vi "configuration UI.vi"() -> ()   [LabVIEW 2013, in "TDMS datalogger editor node.lvclass"]
uses:
  TDMS datalogger editor node.lvclass
  <vilib>/NI/Configuration Framework/Node/NodeRef.ctl
  <vilib>/NI/Configuration Framework/Node/NISE_CEF_Node.lvclass
  <vilib>/NI/AMC/Message Queue.ctl
  <vilib>/NI/AMC/Message.ctl
  <vilib>/NI/Tools/Keyed Array/KeyedArray.ctl
  <vilib>/NI/Configuration Framework/Node/UserEventRef.ctl
  <vilib>/NI/Configuration Framework/Controls/EventCluster.ctl
  module/configuration/TDMS datalogger configuration.lvclass
  <vilib>/NI/Tag Bus Data Framework/Configuration Editor/Classes/Engine Parent/Engine Parent Editor Node.lvclass
  <vilib>/NI/Tag Bus/tag/tag descriptor.lvclass
  <vilib>/NI/Tag Bus/tag/Data Type.ctl
  <vilib>/NI/Module Execution Interface/Engine Configuration/engine configuration.lvclass
  <vilib>/NI/Tag Bus/tag/tag descriptor.lvclass/tag descriptor.ctl
  <vilib>/NI/Configuration Framework/serializable configuration/NISE_CEF_serializable configuration.lvclass/NISE_CEF_serializable configuration.ctl
  <vilib>/NI/Configuration Framework/serializable configuration/NISE_CEF_serializable configuration.lvclass
  module/configuration/TDMS datalogger configuration.lvclass/TDMS datalogger configuration.ctl
  TDMS datalogger editor node.lvclass/TDMS datalogger editor node.ctl
  <vilib>/NI/Tag Bus/tag/write tag name.vi
  <vilib>/NI/Tag Bus/tag/write data type.vi
  module/configuration/Write scans per write.vi
  module/configuration/Write queue size.vi
  module/configuration/Write Path.vi
  module/configuration/Write backup directory.vi
  module/configuration/Write channel pattern matches.vi
  <vilib>/NI/Configuration Framework/serializable configuration/Read UID.vi
  module/configuration/Read backup directory.vi
  module/configuration/Read Path.vi
  module/configuration/Read queue size.vi
  module/configuration/Read scans per write.vi
  module/configuration/Read add enable channel.vi
  module/configuration/Read channel pattern matches.vi
  <vilib>/NI/Tag Bus Data Framework/Configuration Editor/Classes/Module editor node/Read Module Configuration.vi
  <vilib>/NI/Tag Bus Module Framework/module configuration/TBM module configuration.lvclass
  <vilib>/NI/Tag Bus Data Framework/Configuration Editor/Classes/Module editor node/module editor node.lvclass
  <vilib>/NI/Configuration Framework/NISE_CEF_TreeControl.lvlib
  <vilib>/NI/Tools/Keyed Array/Tools_KeyedArray.lvlib
  <vilib>/NI/AMC/AMC.lvlib
panel:
  in  "Tab Control":T1(tab)
  in  "channels":i32(listbox)
  in  "remove":bool
  in  "avail tags":i32(listbox)=-1
  in  "add all":bool
  in  "add1":bool
  out "Enable Tag":string
  in  "history error":bool
  in  "path error":bool
  in  "Historical Directory":path
  in  "use enable channel":bool
  in  "recalc":bool
  out "Approximate memory usage":dbl
  in  "queue size":i32=2
  in  "scans per write":i32=20
  in  "File Path":path
  in  "Channel Subscription Pattern Matches":string[](array[string])
  in  "Enable Dynamic Mapping":bool
  in  "user event":T2
  in  "main queue":T3
  in  "node ref":T4
  # "kB"
  # "Note: This value ignores dynamic mapping"
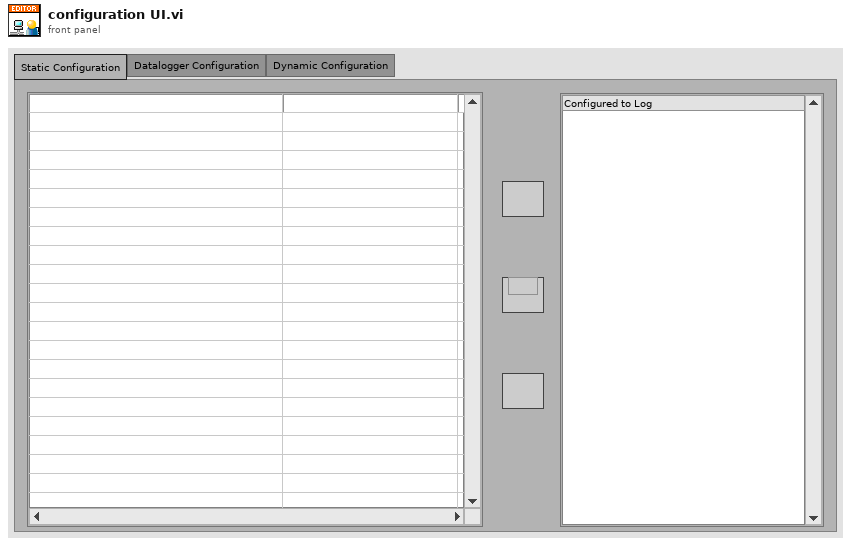
[diagram p1: front panel]
types:
  T1 = enum32{"Static Configuration", "Datalogger Configuration", "Dynamic Configuration"}
  T2 = typedef "NISE_CEF_Node.lvclass/UserEventRef.ctl" = refnum<user-event>
  T3 = typedef "AMC.lvlib/Message Queue.ctl" = refnum<queue>
  T4 = typedef "NISE_CEF_Node.lvclass/NodeRef.ctl" = refnum<data-value>
  T5 = typedef "NISE_CEF_TreeControl.lvlib/EventCluster.ctl" = cluster{"command":string, "data":string}
  T6 = typedef "tag bus.lvlib/tag descriptor.lvclass/Data Type.ctl" = enum16{"Double", "Single", "I64", "I32", "I16", "I8", "U64", "U32", "U16", "U8", "Boolean", "String", "Array of Double", "Array of Single", "Array of I64", "Array of I32", "Array of I16", "Array of I8", "Array of U64", "Array of U32", "Array of U16", "Array of U8", "Array of Boolean", "Array of String"}
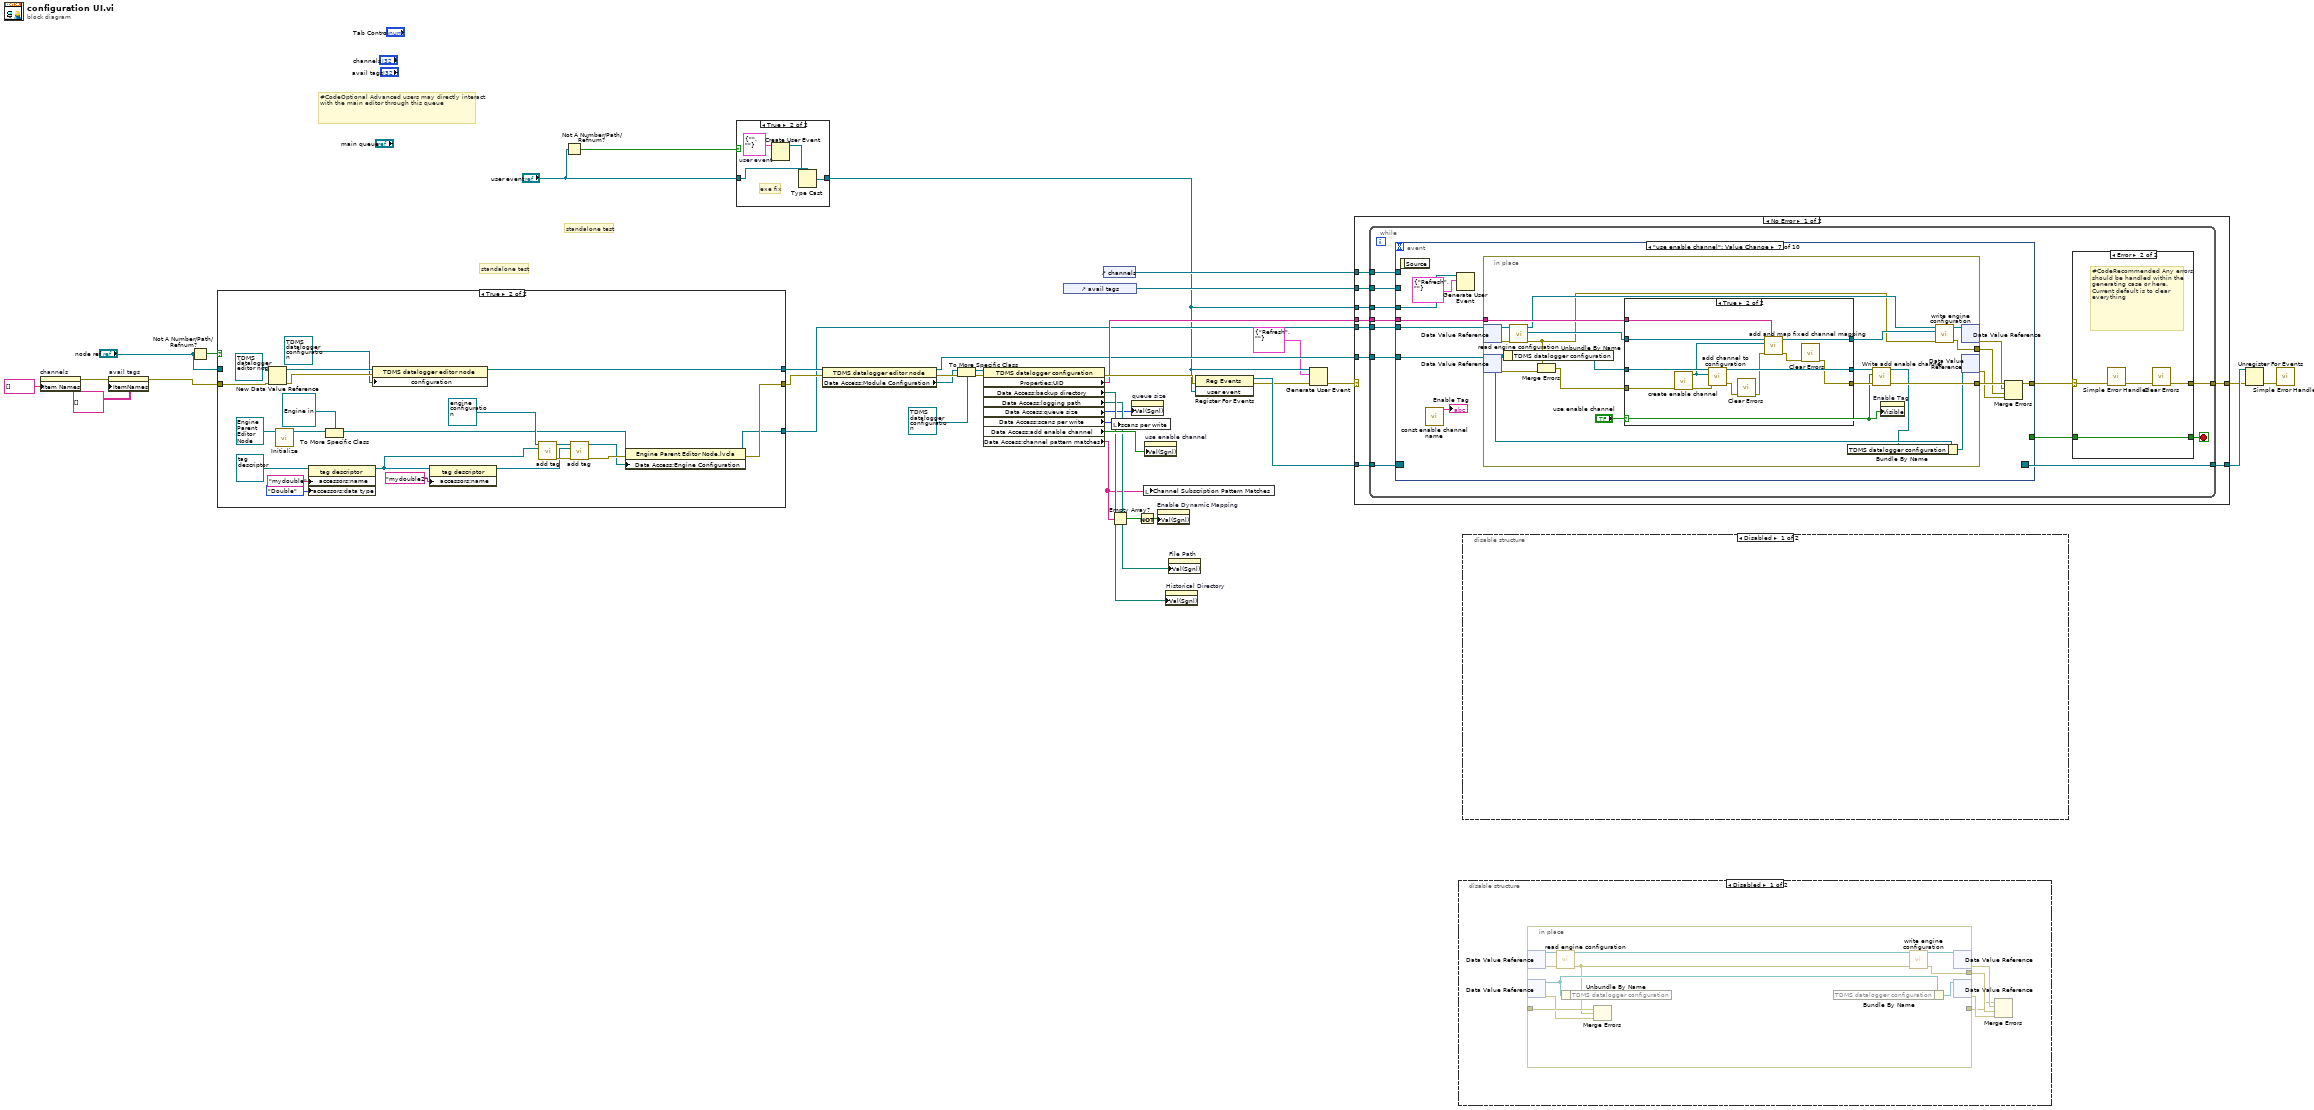
[diagram p0: block diagram]
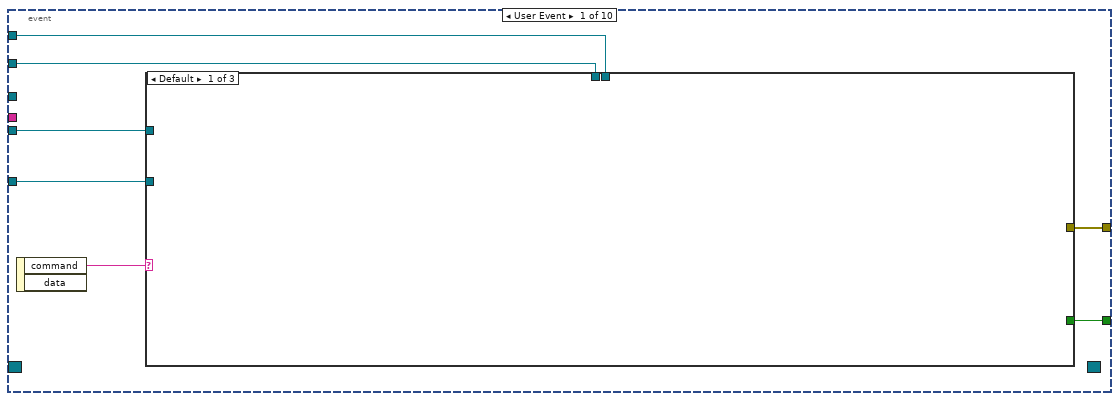
[diagram p4: hidden frame]
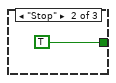
[diagram p5: hidden frame]
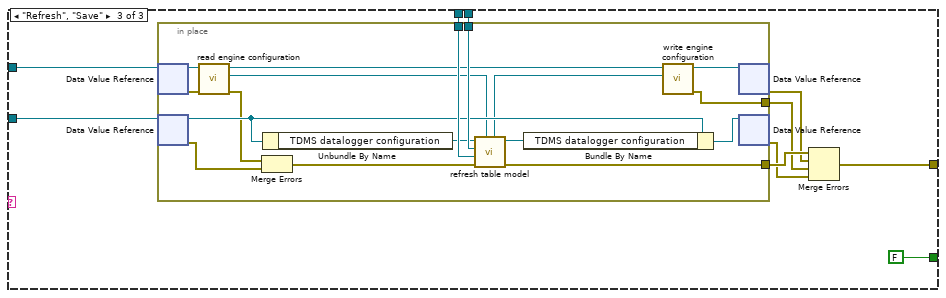
[diagram p6: hidden frame]
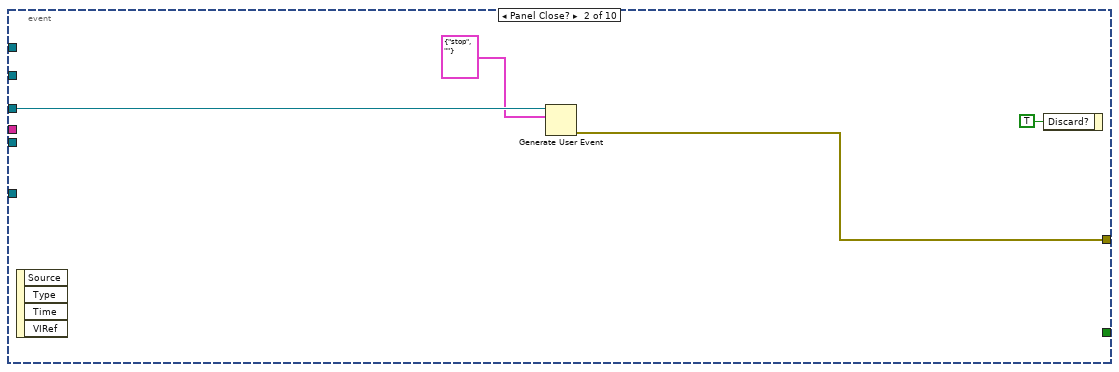
[diagram p7: hidden frame]
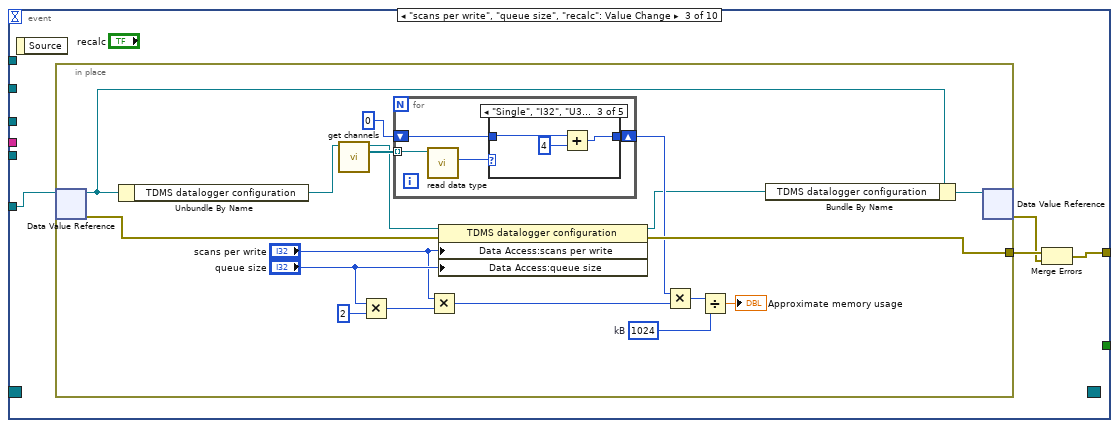
[diagram p8: hidden frame]
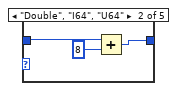
[diagram p10: hidden frame]
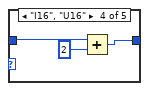
[diagram p11: hidden frame]
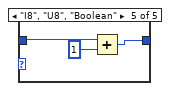
[diagram p12: hidden frame]
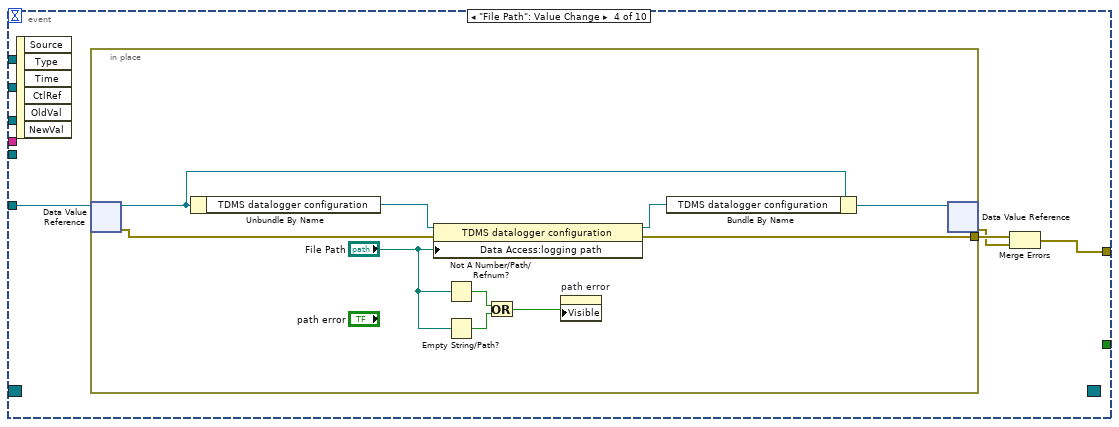
[diagram p13: hidden frame]
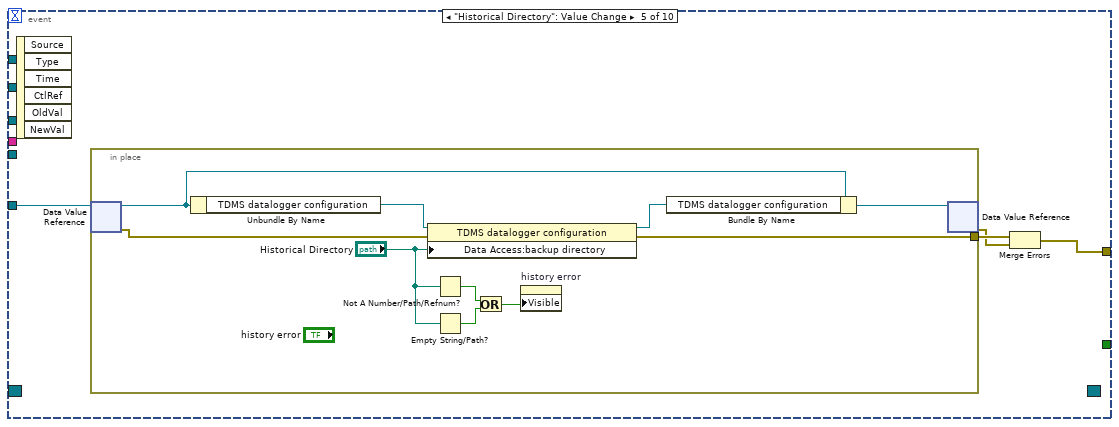
[diagram p14: hidden frame]
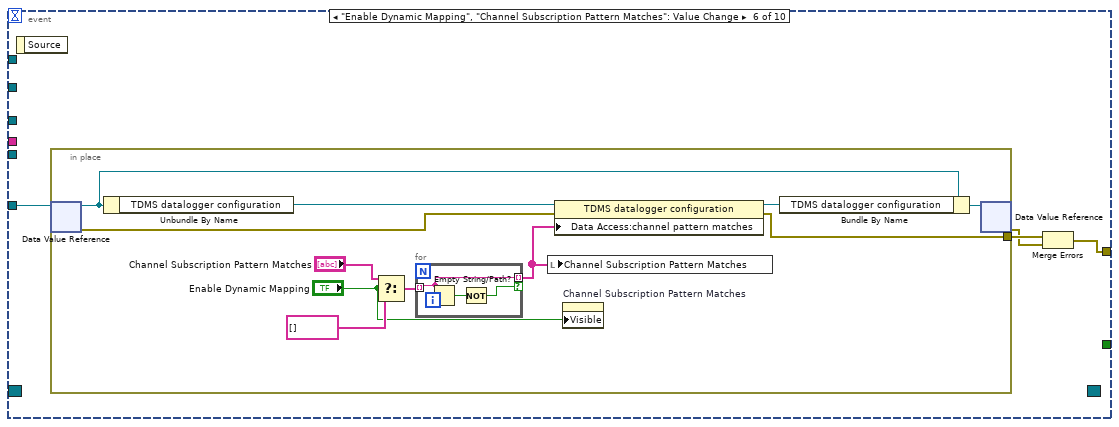
[diagram p15: hidden frame]
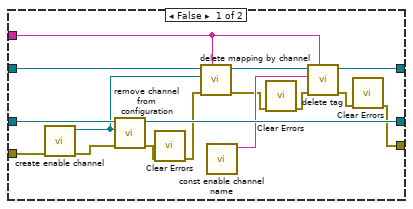
[diagram p16: hidden frame]
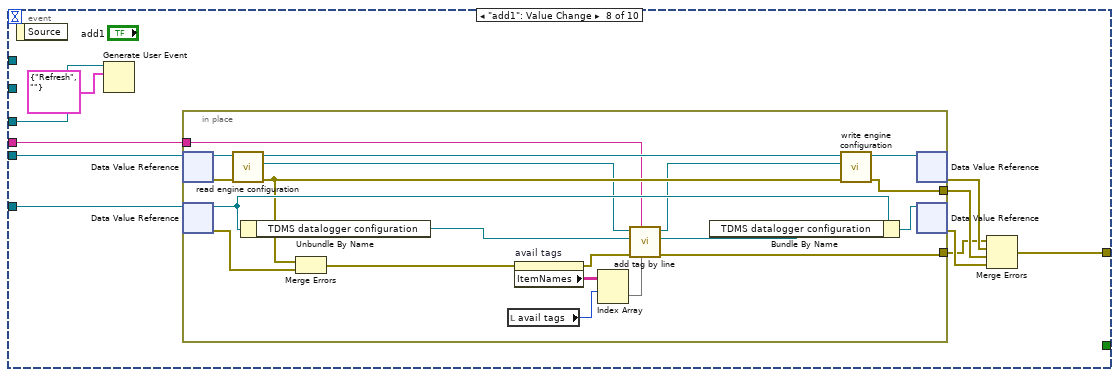
[diagram p17: hidden frame]
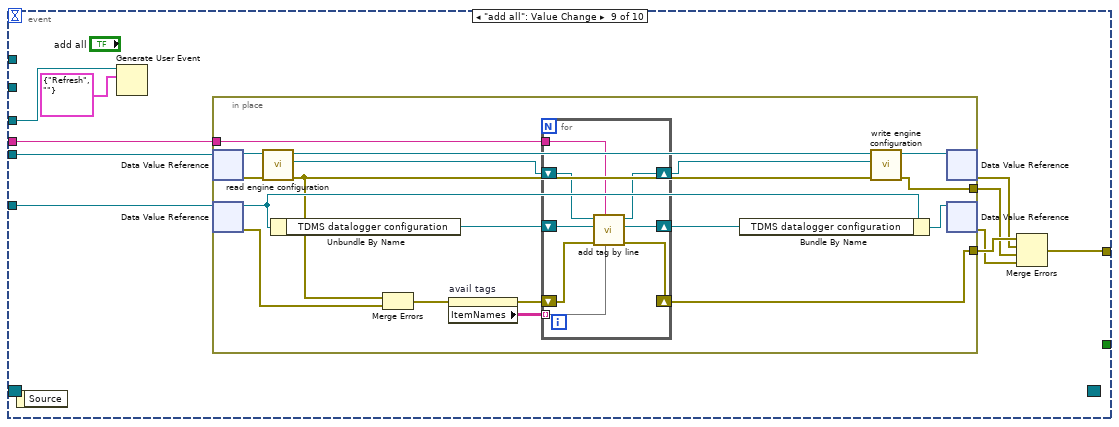
[diagram p18: hidden frame]
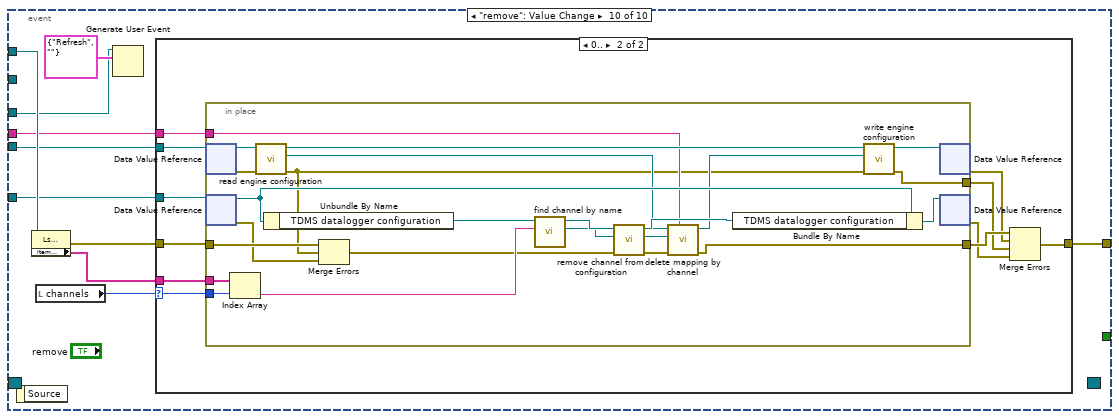
[diagram p19: hidden frame]
diagram:
  # "standalone test"
  # "standalone test"
  # "#CodeOptional Advanced users may directly interact with the main editor through this queue"
  n1 = property on="channels" class="LstBox (strict)"("Item Names"=string[] []) -> (error out=w17:errorcluster)  [unwired: 2 in, 1 out]
  n2 = property on="avail tags" class="MCListbox (strict)"(error in=w17, "ItemNames"=string[][] [] ("Item Names")) -> (error out=w6:errorcluster)  [unwired: 1 in, 1 out]
  n3 = Not A Number/Path/Refnum?(number/path/refnum="node ref") -> (NaN/Path/Refnum?=w8:bool)
  n4 = case shown="True" w8 {
    tunnel: "node ref" -> [w43 _]
    tunnel: [w42 w67] -> w10
    tunnel: [w41 w48] -> w9
    tunnel: [w40 w46] -> w5
    tunnel: w6 -> [w38 w50]
    frame False {
      n5 = call <vilib>:"locate engine.vi"("error in"=w38, "component"=w43) -> ("error out"=w39:errorcluster, "engine"=w40:refnum<data-value>)  [unwired: 8 in]
      n6 = To More Specific Class(target class=refnum<data-value> refnum ("data value reference"), reference=w43, error in=w39) -> (specific class reference=w42:refnum<data-value>, error out=w41:errorcluster)
    }
    frame True {
      n7 = New Data Value Reference(data value=refnum<class "TDMS datalogger editor node.lvclass"> refnum ("tag bus configurable plugin editor node"), error in=w50) -> (data value reference=w66:refnum<data-value>, error out=w51:errorcluster)
      n8 = call-dynamic "Initialize.vi"("Engine in"=refnum<class "Engine Parent Editor Node.lvclass"> refnum) -> ("data value reference"=w65:T4)  [unwired: 8 in, 2 out]
      n9 = property class="tag descriptor"(reference=refnum<class "tag descriptor.lvclass"> refnum ("tag descriptor"), "accessors:name"="mydouble" ("name"), "accessors:data type"=Data_Type."Double" ("data type")) -> (reference out=w54:refnum<class "tag descriptor.lvclass">)  [unwired: 1 in, 1 out]
      n10 = To More Specific Class(target class=refnum<data-value> refnum ("data value reference"), reference=w65) -> (specific class reference=w47:refnum<data-value>)  [unwired: 1 in, 1 out]
      n11 = property class="TDMS datalogger editor node"(reference=w66, error in=w51, "configuration"=refnum<class "TDMS datalogger configuration.lvclass"> refnum ("TDMS datalogger configuration")) -> (reference out=w67:refnum<data-value>)  [unwired: 1 out]
      n12 = property class="tag descriptor"(reference=w54, "accessors:name"="mydouble2" ("name")) -> (reference out=w55:refnum<class "tag descriptor.lvclass">)  [unwired: 1 in, 1 out]
      n13 = call <vilib>:"add tag.vi"("tag descriptor"=w54, "engine configuration in"=refnum<class "engine configuration.lvclass"> refnum ("Engine Configuration")) -> ("error out"=w58:errorcluster, "engine configuration out"=w57:refnum<class "engine configuration.lvclass">)  [unwired: 8 in]
      n14 = call <vilib>:"add tag.vi"("error in"=w58, "tag descriptor"=w55, "engine configuration in"=w57) -> ("error out"=w56:errorcluster, "engine configuration out"=w45:refnum<class "engine configuration.lvclass">)  [unwired: 7 in]
      n15 = property class="Engine Parent Editor Node.lvcla"(reference=w47, error in=w56, "Data Access:Engine Configuration"=w45) -> (reference out=w46:refnum<data-value>, error out=w48:errorcluster)
    }
  }
  n16 = Not A Number/Path/Refnum?(number/path/refnum="user event") -> (NaN/Path/Refnum?=w12:bool)
  n17 = case shown="True" w12 {
    tunnel: [w68 w71] -> w4
    tunnel: "user event" -> [w68 w72]
    frame False {
    }
    frame True {
      w69 = T5 {"command"="", "data"=""}  # user event
      # "exe fix"
      n18 = Create User Event(user event datatype=w69) -> (user event=w70:refnum<user-event>)  [unwired: 1 in, 1 out]
      n19 = Type Cast(type=w72, x=w70) -> (*(type *) &x=w71:T2)
    }
  }
  n20 = property class="TDMS datalogger editor node"(reference=w10, error in=w9) -> (reference out=w13:refnum<data-value>, error out=w34:errorcluster, "Data Access:Module Configuration"=w24:refnum<class "TBM module configuration.lvclass">)
  n21 = To More Specific Class(target class=refnum<class "TDMS datalogger configuration.lvclass"> refnum ("TDMS datalogger configuration"), reference=w24, error in=w34) -> (specific class reference=w22:refnum<class "TDMS datalogger configuration.lvclass">, error out=w25:errorcluster)
  n22 = property class="TDMS datalogger configuration"(reference=w22, error in=w25) -> (error out=w21:errorcluster, "Properties:UID"=w18:string, "Data Access:backup directory"=w31:path, "Data Access:logging path"=w30:path, "Data Access:queue size"=w29:i32, "Data Access:scans per write"=w33:i32, "Data Access:add enable channel"=w32:bool, "Data Access:channel pattern matches"=w28:string[])  [unwired: 1 out]
  n23 = control-ref of="avail tags"() -> (w19:refnum<vi>)
  n24 = control-ref of="channels"() -> (w20:refnum<vi>)
  n25 = Empty Array?(array=w28) -> (empty?=w26:bool)
  n26 = local write "scans per write"(w33) -> ()
  n27 = property on="queue size" class="DigNum (strict)"("Val(Sgnl)"=w29) -> ()  [unwired: 2 in, 2 out]
  n28 = Not(x=w26) -> (.not. x?=w27:bool)
  n29 = local write "Channel Subscription Pattern Matches"(w28) -> ()
  n30 = property on="use enable channel" class="Bool (strict)"("Val(Sgnl)"=w32) -> ()  [unwired: 2 in, 2 out]
  n31 = property on="Enable Dynamic Mapping" class="Bool (strict)"("Val(Sgnl)"=w27) -> ()  [unwired: 2 in, 2 out]
  n32 = property on="Historical Directory" class="Path"("Val(Sgnl)"=w31) -> ()  [unwired: 2 in, 2 out]
  n33 = property on="File Path" class="Path"("Val(Sgnl)"=w30) -> ()  [unwired: 2 in, 2 out]
  n34 = register-events(error in=w21, w4) -> (reference out=w37:refnum<event-registration>, error out=w2:errorcluster)  [unwired: 1 in]
  n35 = Generate User Event(user event=w4, event data cluster=T5 {"command"="Refresh", "data"=""} ("event data"), error in=w2) -> (error out=w1:errorcluster)  [unwired: 1 in, 1 out]
  n36 = case shown="No Error" w1 {
    selector: w1 -> [_ w394]
    tunnel: w37 -> [w81 w393]
    tunnel: [w80 w393] -> w36
    tunnel: w20 -> [w79 _]
    tunnel: w19 -> [w78 _]
    tunnel: w18 -> [w77 _]
    tunnel: [w76 w394] -> w14
    tunnel: w13 -> [w75 _]
    tunnel: w5 -> [w74 _]
    tunnel: w4 -> [w73 _]
    frame No Error {
      n37 = while {
        tunnel: w81 -> [w93]
        tunnel: [w92] -> w80
        tunnel: w79 -> [w88]
        tunnel: w78 -> [w87]
        tunnel: w77 -> [w82]
        tunnel: w74 -> [w86]
        tunnel: w75 -> [w85]
        tunnel: w73 -> [w84]
        tunnel: [w89] -> w76
        stop <- w90 stop-if-true
        n38 = event shown="[6] \"use enable channel\": Value Change" {
          selector: w93 -> [_ _ _ _ _ _ _ _ _ _]
          dyn-events: [_ _ _ _ _ _ _ _ _ _] -> w92
          timeout: _ -> [_ _ _ _ _ _ _ _ _ _]
          tunnel: [w106 _ _ _ _ _ _ _ _ _] -> w83
          tunnel: [w104 w137 w140 w180 w194 w206 w230 w283 w315 w357] -> w91
          tunnel: w88 -> [w101 _ _ _ _ _ _ _ _ w355]
          tunnel: w87 -> [w100 _ _ _ _ _ _ _ _ _]
          tunnel: w86 -> [w103 _ _ _ _ _ w228 w284 w313 w348]
          tunnel: w85 -> [w102 _ w141 w179 w193 w207 w229 w285 w314 w349]
          tunnel: w84 -> [_ w136 _ _ _ _ w232 w290 w320 w350]
          tunnel: w82 -> [_ _ _ _ _ _ w234 w282 w312 w353]
          event User Event {
            n39 = event-data() -> ("command"=w105:string)  [unwired: 1 in, 1 out]
            n40 = case shown="Default" w105 {
              tunnel: [_ TRUE FALSE] -> w106
              tunnel: [_ _ w113] -> w104
              tunnel: w103 -> [_ _ w112]
              tunnel: w102 -> [_ _ w111]
              tunnel: w101 -> [_ _ w115]
              tunnel: w100 -> [_ _ w114]
              frame Default {
              }
              frame "Stop" {
              }
              frame "Refresh", "Save" {
                n41 = in-place {
                  in-place-border: [w134] -> w116
                  in-place-border: w115 -> [w133]
                  in-place-border: w114 -> [w132]
                  in-place-border: [w118] -> w110
                  n42 = in-place-dvr #1(w112) -> (w122:refnum<class "Engine Parent Editor Node.lvclass">, w123:errorcluster)
                  n43 = in-place-dvr #2(w111) -> (w129:refnum<class "TDMS datalogger editor node.lvclass">, w126:errorcluster)
                  n44 = call <vilib>:"read engine configuration.vi"("error in"=w123, "Engine Parent Editor Node in"=w122) -> ("error out"=w119:errorcluster, "engine configuration"=w120:refnum<class "engine configuration.lvclass">, "Engine Parent Editor Node out"=w121:refnum<class "Engine Parent Editor Node.lvclass">)  [unwired: 7 in]
                  n45 = Merge Errors(w119, w126) -> (w131:errorcluster)
                  n46 = Unbundle By Name(w129) -> ("TDMS datalogger configuration"=w130:refnum<class "TDMS datalogger configuration.lvclass">)
                  n47 = call "refresh table model.vi"("engine configuration"=w120, "error in"=w131, "avail tags"=w132, "chan table"=w133, "TDMS datalogger configuration"=w130) -> ("error out"=w134:errorcluster, "TDMS datalogger configuration out"=w127:refnum<class "TDMS datalogger configuration.lvclass">, "engine configuration out"=w124:refnum<class "engine configuration.lvclass">)  [unwired: 4 in]
                  n48 = Bundle By Name(cluster=w129, "TDMS datalogger configuration"=w127) -> (w128:refnum<class "TDMS datalogger editor node.lvclass">)
                  n49 = call <vilib>:"write engine configuration.vi"("engine configuration"=w124, "Engine Parent Editor Node in"=w121) -> ("error out"=w118:errorcluster, "Engine Parent Editor Node out"=w125:refnum<class "Engine Parent Editor Node.lvclass">)  [unwired: 8 in]
                  n50 = in-place-dvr #1(w125) -> (w109:errorcluster)  [unwired: 1 out]
                  n51 = in-place-dvr #2(w128) -> (w108:errorcluster)  [unwired: 1 out]
                }
                n52 = Merge Errors(w116, w109, w110, w108) -> (w113:errorcluster)
              }
            }
          }
          event Panel Close? {
            n53 = event-data() -> ()  [unwired: 1 in, 4 out]
            n54 = Generate User Event(user event=w136, event data cluster=T5 {"command"="stop", "data"=""} ("event data")) -> (error out=w137:errorcluster)  [unwired: 2 in, 1 out]
            n55 = event-data("Discard?"=TRUE) -> ()  [unwired: 1 in, 1 out]
          }
          event "scans per write", "queue size", "recalc": Value Change {
            n56 = event-data() -> ()  [unwired: 1 in, 1 out]
            n57 = in-place {
              in-place-border: [w160] -> w142
              w154 = u32 1024  # kB
              n58 = in-place-dvr #3(w141) -> (w146:refnum<class "TDMS datalogger editor node.lvclass">, w147:errorcluster)
              n59 = Unbundle By Name(w146) -> ("TDMS datalogger configuration"=w144:refnum<class "TDMS datalogger configuration.lvclass">)
              n60 = call-dynamic "get channels.vi"("module configuration in"=w144) -> ("channels"=w150:refnum<class "TBM channel.lvclass">[], "module configuration out"=w148:refnum<class "TDMS datalogger configuration.lvclass">)  [unwired: 9 in]
              n61 = Multiply(x="queue size", y=2 ("x")) -> (x*y=w159:i32)
              n62 = for {
                shift-right: [w163] -> w151
                shift-left: u32 0 -> [w164]
                tunnel: w150 -> [w161] mode=indexing
                n63 = call <vilib>:"read data type.vi"("system tag in"=w161) -> ("data type"=w162:T6)  [unwired: 8 in, 2 out]
                n64 = case shown="\"Single\", \"I32\", \"U32\"" w162 {
                  tunnel: w164 -> [w165 w168 w171 w174 w177]
                  tunnel: [w165 w167 w170 w173 w176] -> w163
                  frame Default {
                  }
                  frame "Double", "I64", "U64" {
                    n65 = Add(x=w168, y=u32 8) -> (x+y=w167:u32)
                  }
                  frame "Single", "I32", "U32" {
                    n66 = Add(x=w171, y=u32 4) -> (x+y=w170:u32)
                  }
                  frame "I16", "U16" {
                    n67 = Add(x=w174, y=u32 2) -> (x+y=w173:u32)
                  }
                  frame "I8", "U8", "Boolean" {
                    n68 = Add(x=w177, y=u32 1) -> (x+y=w176:u32)
                  }
                }
              }
              n69 = Multiply(x="scans per write", y=w159) -> (x*y=w153:i32)
              n70 = property class="TDMS datalogger configuration"(reference=w148, error in=w147, "Data Access:scans per write"="scans per write", "Data Access:queue size"="queue size") -> (reference out=w143:refnum<class "TDMS datalogger configuration.lvclass">, error out=w160:errorcluster)
              n71 = Multiply(x=w151, y=w153) -> (x*y=w155:u32)
              n72 = Divide(x=w155, y=w154) -> (x/y=→"Approximate memory usage":dbl)
              n73 = Bundle By Name(cluster=w146, "TDMS datalogger configuration"=w143) -> (w145:refnum<class "TDMS datalogger editor node.lvclass">)
              n74 = in-place-dvr #3(w145) -> (w139:errorcluster)  [unwired: 1 out]
            }
            n75 = Merge Errors(w142, w139) -> (w140:errorcluster)
          }
          event "File Path": Value Change {
            n76 = event-data() -> ()  [unwired: 1 in, 6 out]
            n77 = in-place {
              in-place-border: [w191] -> w181
              n78 = in-place-dvr #4(w179) -> (w182:refnum<class "TDMS datalogger editor node.lvclass">, w185:errorcluster)
              n79 = Unbundle By Name(w182) -> ("TDMS datalogger configuration"=w186:refnum<class "TDMS datalogger configuration.lvclass">)
              n80 = property class="TDMS datalogger configuration"(reference=w186, error in=w185, "Data Access:logging path"="File Path") -> (reference out=w184:refnum<class "TDMS datalogger configuration.lvclass">, error out=w191:errorcluster)
              n81 = Not A Number/Path/Refnum?(number/path/refnum="File Path") -> (NaN/Path/Refnum?=w188:bool)
              n82 = Empty String/Path?(string/path="File Path") -> (empty?=w189:bool)
              n83 = Or(x=w188, y=w189) -> (x .or. y?=w187:bool)
              n84 = property on="path error" class="Bool"("Visible"=w187) -> ()  [unwired: 2 in, 2 out]
              n85 = Bundle By Name(cluster=w182, "TDMS datalogger configuration"=w184) -> (w183:refnum<class "TDMS datalogger editor node.lvclass">)
              n86 = in-place-dvr #4(w183) -> (w178:errorcluster)  [unwired: 1 out]
            }
            n87 = Merge Errors(w181, w178) -> (w180:errorcluster)
          }
          event "Historical Directory": Value Change {
            n88 = event-data() -> ()  [unwired: 1 in, 6 out]
            n89 = in-place {
              in-place-border: [w199] -> w195
              n90 = in-place-dvr #5(w193) -> (w204:refnum<class "TDMS datalogger editor node.lvclass">, w196:errorcluster)
              n91 = Unbundle By Name(w204) -> ("TDMS datalogger configuration"=w197:refnum<class "TDMS datalogger configuration.lvclass">)
              n92 = property class="TDMS datalogger configuration"(reference=w197, error in=w196, "Data Access:backup directory"="Historical Directory") -> (reference out=w198:refnum<class "TDMS datalogger configuration.lvclass">, error out=w199:errorcluster)
              n93 = Not A Number/Path/Refnum?(number/path/refnum="Historical Directory") -> (NaN/Path/Refnum?=w202:bool)
              n94 = Empty String/Path?(string/path="Historical Directory") -> (empty?=w203:bool)
              n95 = Or(x=w202, y=w203) -> (x .or. y?=w200:bool)
              n96 = property on="history error" class="Bool"("Visible"=w200) -> ()  [unwired: 2 in, 2 out]
              n97 = Bundle By Name(cluster=w204, "TDMS datalogger configuration"=w198) -> (w205:refnum<class "TDMS datalogger editor node.lvclass">)
              n98 = in-place-dvr #5(w205) -> (w192:errorcluster)  [unwired: 1 out]
            }
            n99 = Merge Errors(w195, w192) -> (w194:errorcluster)
          }
          event "Enable Dynamic Mapping", "Channel Subscription Pattern Matches": Value Change {
            n100 = event-data() -> ()  [unwired: 1 in, 1 out]
            n101 = in-place {
              in-place-border: [w210] -> w209
              n102 = in-place-dvr #6(w207) -> (w219:refnum<class "TDMS datalogger editor node.lvclass">, w211:errorcluster)
              n103 = Unbundle By Name(w219) -> ("TDMS datalogger configuration"=w212:refnum<class "TDMS datalogger configuration.lvclass">)
              n104 = Select(t="Channel Subscription Pattern Matches", s="Enable Dynamic Mapping", f=string[] []) -> (s? t:f=w215:string[])
              n105 = for {
                tunnel: w215 -> [w223] mode=indexing
                tunnel: [w223] -> w214 mode=indexing if=w221
                n106 = Empty String/Path?(string/path=w223) -> (empty?=w222:bool)
                n107 = Not(x=w222) -> (.not. x?=w221:bool)
              }
              n108 = local write "Channel Subscription Pattern Matches"(w214) -> ()
              n109 = property class="TDMS datalogger configuration"(reference=w212, error in=w211, "Data Access:channel pattern matches"=w214) -> (reference out=w213:refnum<class "TDMS datalogger configuration.lvclass">, error out=w210:errorcluster)
              n110 = property on="Channel Subscription Pattern Matches" class="Arr (strict)"("Visible"="Enable Dynamic Mapping") -> ()  [unwired: 2 in, 2 out]
              n111 = Bundle By Name(cluster=w219, "TDMS datalogger configuration"=w213) -> (w220:refnum<class "TDMS datalogger editor node.lvclass">)
              n112 = in-place-dvr #6(w220) -> (w208:errorcluster)  [unwired: 1 out]
            }
            n113 = Merge Errors(w209, w208) -> (w206:errorcluster)
          }
          event "use enable channel": Value Change {
            n114 = event-data() -> ()  [unwired: 1 in, 1 out]
            n115 = call "const enable channel name.vi"() -> ("enable channel"=→"Enable Tag":string)  [unwired: 11 in]
            n116 = Generate User Event(user event=w232, event data cluster=T5 {"command"="Refresh", "data"=""} ("event data")) -> ()  [unwired: 2 in, 2 out]
            n117 = in-place {
              in-place-border: w234 -> [w253]
              in-place-border: [w250] -> w231
              in-place-border: [w244] -> w226
              n118 = in-place-dvr #7(w228) -> (w248:refnum<class "Engine Parent Editor Node.lvclass">, w246:errorcluster)
              n119 = in-place-dvr #8(w229) -> (w242:refnum<class "TDMS datalogger editor node.lvclass">, w245:errorcluster)
              n120 = Unbundle By Name(w242) -> ("TDMS datalogger configuration"=w243:refnum<class "TDMS datalogger configuration.lvclass">)
              n121 = call <vilib>:"read engine configuration.vi"("error in"=w246, "Engine Parent Editor Node in"=w248) -> ("error out"=w236:errorcluster, "engine configuration"=w247:refnum<class "engine configuration.lvclass">, "Engine Parent Editor Node out"=w238:refnum<class "Engine Parent Editor Node.lvclass">)  [unwired: 7 in]
              n122 = Merge Errors(w236, w245) -> (w235:errorcluster)
              n123 = case shown="True" "use enable channel" {
                tunnel: w253 -> [w262 w280]
                tunnel: [w263 w281] -> w237
                tunnel: w247 -> [w266 w275]
                tunnel: [w268 w279] -> w252
                tunnel: w243 -> [w269 w278]
                tunnel: [w257 w273] -> w251
                tunnel: w235 -> [w254 w270]
                frame False {
                  n124 = call "create enable channel.vi"("error in"=w254) -> ("error out"=w267:errorcluster, "enable channel"=w265:refnum<class "TBM channel.lvclass">)  [unwired: 9 in]
                  n125 = call "remove channel from configuration.vi"("error in"=w267, "TBM channel in"=w265, "TDMS datalogger configuration in"=w269) -> ("error out"=w256:errorcluster, "TDMS datalogger configuration out"=w268:refnum<class "TDMS datalogger configuration.lvclass">)  [unwired: 7 in]
                  n126 = call <vilib>:"Clear Errors.vi"("error in (no error)"=w256) -> ("error out"=w255:errorcluster)  [unwired: 6 in]
                  n127 = call <vilib>:"delete mapping by channel.vi"("owner ID"=w262, "error in"=w255, "channel"=w265, "engine configuration in"=w266) -> ("error out"=w259:errorcluster, "engine configuration out"=w264:refnum<class "engine configuration.lvclass">)  [unwired: 6 in]
                  n128 = call "const enable channel name.vi"() -> ("enable channel"=w261:string)  [unwired: 11 in]
                  n129 = call <vilib>:"Clear Errors.vi"("error in (no error)"=w259) -> ("error out"=w260:errorcluster)  [unwired: 6 in]
                  n130 = call <vilib>:"delete tag.vi"("owner ID"=w262, "error in"=w260, "tag name"=w261, "engine configuration in"=w264) -> ("error out"=w258:errorcluster, "engine configuration out"=w263:refnum<class "engine configuration.lvclass">)  [unwired: 6 in]
                  n131 = call <vilib>:"Clear Errors.vi"("error in (no error)"=w258) -> ("error out"=w257:errorcluster)  [unwired: 6 in]
                }
                frame True {
                  n132 = call "create enable channel.vi"("error in"=w270) -> ("error out"=w277:errorcluster, "enable channel"=w276:refnum<class "TBM channel.lvclass">)  [unwired: 9 in]
                  n133 = call "add channel to configuration.vi"("error in"=w277, "TBM channel in"=w276, "TDMS datalogger configuration in"=w278) -> ("error out"=w272:errorcluster, "TDMS datalogger configuration out"=w279:refnum<class "TDMS datalogger configuration.lvclass">)  [unwired: 7 in]
                  n134 = call <vilib>:"Clear Errors.vi"("error in (no error)"=w272) -> ("error out"=w271:errorcluster)  [unwired: 6 in]
                  n135 = call <vilib>:"add and map fixed channel mapping.vi"("module instance"=w280, "error in"=w271, "fixed channel"=w276, "engine configuration in"=w275) -> ("error out"=w274:errorcluster, "engine configuration out"=w281:refnum<class "engine configuration.lvclass">)  [unwired: 6 in]
                  n136 = call <vilib>:"Clear Errors.vi"("error in (no error)"=w274) -> ("error out"=w273:errorcluster)  [unwired: 6 in]
                }
              }
              n137 = call "Write add enable channel.vi"("error in (no error)"=w251, "add enable channel"="use enable channel", "TDMS datalogger configuration in"=w252) -> ("error out"=w250:errorcluster, "TDMS datalogger configuration out"=w241:refnum<class "TDMS datalogger configuration.lvclass">)  [unwired: 7 in]
              n138 = Bundle By Name(cluster=w242, "TDMS datalogger configuration"=w241) -> (w240:refnum<class "TDMS datalogger editor node.lvclass">)
              n139 = property on="Enable Tag" class="Str"("Visible"="use enable channel") -> ()  [unwired: 2 in, 2 out]
              n140 = call <vilib>:"write engine configuration.vi"("error in"=w236, "engine configuration"=w237, "Engine Parent Editor Node in"=w238) -> ("error out"=w244:errorcluster, "Engine Parent Editor Node out"=w239:refnum<class "Engine Parent Editor Node.lvclass">)  [unwired: 7 in]
              n141 = in-place-dvr #7(w239) -> (w227:errorcluster)  [unwired: 1 out]
              n142 = in-place-dvr #8(w240) -> (w225:errorcluster)  [unwired: 1 out]
            }
            n143 = Merge Errors(w231, w227, w226, w225) -> (w230:errorcluster)
          }
          event "add1": Value Change {
            n144 = event-data() -> ()  [unwired: 1 in, 1 out]
            n145 = Generate User Event(user event=w290, event data cluster=T5 {"command"="Refresh", "data"=""} ("event data")) -> ()  [unwired: 2 in, 2 out]
            n146 = in-place {
              in-place-border: [w296] -> w286
              in-place-border: [w305] -> w287
              in-place-border: w282 -> [w292]
              n147 = in-place-dvr #9(w284) -> (w307:refnum<class "Engine Parent Editor Node.lvclass">, w308:errorcluster)
              n148 = in-place-dvr #10(w285) -> (w304:refnum<class "TDMS datalogger editor node.lvclass">, w310:errorcluster)
              n149 = call <vilib>:"read engine configuration.vi"("error in"=w308, "Engine Parent Editor Node in"=w307) -> ("error out"=w303:errorcluster, "engine configuration"=w294:refnum<class "engine configuration.lvclass">, "Engine Parent Editor Node out"=w306:refnum<class "Engine Parent Editor Node.lvclass">)  [unwired: 7 in]
              n150 = Unbundle By Name(w304) -> ("TDMS datalogger configuration"=w298:refnum<class "TDMS datalogger configuration.lvclass">)
              n151 = Merge Errors(w303, w310) -> (w293:errorcluster)
              n152 = local read "avail tags"() -> (w300:i32)
              n153 = property on="avail tags" class="MCListbox (strict)"(error in=w293) -> (error out=w301:errorcluster, "ItemNames"=w299:string[][])  [unwired: 1 in, 1 out]
              n154 = Index Array(array=w299, index (row)=w300) -> (element=w302:string[])  [unwired: 1 in]
              n155 = call "add tag by line.vi"("ItemNames"=w302, "Properties:instance identifier"=w292, "error in"=w301, "TDMS datalogger configuration in"=w298, "engine configuration in"=w294) -> ("error out"=w296:errorcluster, "TDMS datalogger configuration out"=w297:refnum<class "TDMS datalogger configuration.lvclass">, "engine configuration out"=w295:refnum<class "engine configuration.lvclass">)  [unwired: 4 in]
              n156 = Bundle By Name(cluster=w304, "TDMS datalogger configuration"=w297) -> (w311:refnum<class "TDMS datalogger editor node.lvclass">)
              n157 = call <vilib>:"write engine configuration.vi"("error in"=w303, "engine configuration"=w295, "Engine Parent Editor Node in"=w306) -> ("error out"=w305:errorcluster, "Engine Parent Editor Node out"=w309:refnum<class "Engine Parent Editor Node.lvclass">)  [unwired: 7 in]
              n158 = in-place-dvr #9(w309) -> (w288:errorcluster)  [unwired: 1 out]
              n159 = in-place-dvr #10(w311) -> (w289:errorcluster)  [unwired: 1 out]
            }
            n160 = Merge Errors(w286, w288, w287, w289) -> (w283:errorcluster)
          }
          event "add all": Value Change {
            n161 = event-data() -> ()  [unwired: 1 in, 1 out]
            n162 = Generate User Event(user event=w320, event data cluster=T5 {"command"="Refresh", "data"=""} ("event data")) -> ()  [unwired: 2 in, 2 out]
            n163 = in-place {
              in-place-border: [w324] -> w319
              in-place-border: [w333] -> w318
              in-place-border: w312 -> [w322]
              n164 = in-place-dvr #11(w313) -> (w335:refnum<class "Engine Parent Editor Node.lvclass">, w336:errorcluster)
              n165 = in-place-dvr #12(w314) -> (w332:refnum<class "TDMS datalogger editor node.lvclass">, w338:errorcluster)
              n166 = call <vilib>:"read engine configuration.vi"("error in"=w336, "Engine Parent Editor Node in"=w335) -> ("error out"=w331:errorcluster, "engine configuration"=w326:refnum<class "engine configuration.lvclass">, "Engine Parent Editor Node out"=w334:refnum<class "Engine Parent Editor Node.lvclass">)  [unwired: 7 in]
              n167 = Unbundle By Name(w332) -> ("TDMS datalogger configuration"=w327:refnum<class "TDMS datalogger configuration.lvclass">)
              n168 = Merge Errors(w331, w338) -> (w323:errorcluster)
              n169 = property on="avail tags" class="MCListbox (strict)"(error in=w323) -> (error out=w329:errorcluster, "ItemNames"=w330:string[][])  [unwired: 1 in, 1 out]
              n170 = for {
                tunnel: w330 -> [w341] mode=indexing
                shift-right: [w346] -> w324
                shift-left: w329 -> [w344]
                shift-right: [w347] -> w328
                shift-left: w327 -> [w345]
                shift-right: [w342] -> w325
                shift-left: w326 -> [w343]
                tunnel: w322 -> [w340]
                n171 = call "add tag by line.vi"("ItemNames"=w341, "Properties:instance identifier"=w340, "error in"=w344, "TDMS datalogger configuration in"=w345, "engine configuration in"=w343) -> ("error out"=w346:errorcluster, "TDMS datalogger configuration out"=w347:refnum<class "TDMS datalogger configuration.lvclass">, "engine configuration out"=w342:refnum<class "engine configuration.lvclass">)  [unwired: 4 in]
              }
              n172 = Bundle By Name(cluster=w332, "TDMS datalogger configuration"=w328) -> (w339:refnum<class "TDMS datalogger editor node.lvclass">)
              n173 = call <vilib>:"write engine configuration.vi"("error in"=w331, "engine configuration"=w325, "Engine Parent Editor Node in"=w334) -> ("error out"=w333:errorcluster, "Engine Parent Editor Node out"=w337:refnum<class "Engine Parent Editor Node.lvclass">)  [unwired: 7 in]
              n174 = in-place-dvr #11(w337) -> (w317:errorcluster)  [unwired: 1 out]
              n175 = in-place-dvr #12(w339) -> (w316:errorcluster)  [unwired: 1 out]
            }
            n176 = Merge Errors(w319, w317, w318, w316) -> (w315:errorcluster)
          }
          event "remove": Value Change {
            n177 = event-data() -> ()  [unwired: 1 in, 1 out]
            n178 = property class="LstBox (strict)"(reference=w355) -> (error out=w354:errorcluster, "Item Names"=w356:string[])  [unwired: 1 in, 1 out]
            n179 = local read "channels"() -> (w352:i32)
            n180 = Generate User Event(user event=w350, event data cluster=T5 {"command"="Refresh", "data"=""} ("event data")) -> ()  [unwired: 2 in, 2 out]
            n181 = case shown="0.." w352 {
              selector: w352 -> [_ w360]
              tunnel: [w358 w365] -> w357
              tunnel: w356 -> [_ w361]
              tunnel: w354 -> [w358 w362]
              tunnel: w353 -> [_ w359]
              tunnel: w349 -> [_ w364]
              tunnel: w348 -> [_ w363]
              frame ..-1 {
              }
              frame 0.. {
                n182 = in-place {
                  in-place-border: w362 -> [w392]
                  in-place-border: [w372] -> w369
                  in-place-border: [w385] -> w368
                  in-place-border: w361 -> [w376]
                  in-place-border: w360 -> [w375]
                  in-place-border: w359 -> [w374]
                  n183 = in-place-dvr #13(w363) -> (w387:refnum<class "Engine Parent Editor Node.lvclass">, w388:errorcluster)
                  n184 = in-place-dvr #14(w364) -> (w384:refnum<class "TDMS datalogger editor node.lvclass">, w390:errorcluster)
                  n185 = Index Array(array=w376, index=w375) -> (element=w381:string)
                  n186 = call <vilib>:"read engine configuration.vi"("error in"=w388, "Engine Parent Editor Node in"=w387) -> ("error out"=w370:errorcluster, "engine configuration"=w373:refnum<class "engine configuration.lvclass">, "Engine Parent Editor Node out"=w386:refnum<class "Engine Parent Editor Node.lvclass">)  [unwired: 7 in]
                  n187 = Unbundle By Name(w384) -> ("TDMS datalogger configuration"=w378:refnum<class "TDMS datalogger configuration.lvclass">)
                  n188 = Merge Errors(w392, w370, w390) -> (w377:errorcluster)
                  n189 = call "find channel by name.vi"("channel name"=w381, "TDMS datalogger configuration in"=w378) -> ("channel"=w380:refnum<class "TBM channel.lvclass">, "TDMS datalogger configuration out"=w382:refnum<class "TDMS datalogger configuration.lvclass">)  [unwired: 8 in]
                  n190 = call "remove channel from configuration.vi"("error in"=w377, "TBM channel in"=w380, "TDMS datalogger configuration in"=w382) -> ("error out"=w383:errorcluster, "TDMS datalogger configuration out"=w379:refnum<class "TDMS datalogger configuration.lvclass">)  [unwired: 7 in]
                  n191 = call <vilib>:"delete mapping by channel.vi"("owner ID"=w374, "error in"=w383, "channel"=w380, "engine configuration in"=w373) -> ("error out"=w372:errorcluster, "engine configuration out"=w371:refnum<class "engine configuration.lvclass">)  [unwired: 6 in]
                  n192 = Bundle By Name(cluster=w384, "TDMS datalogger configuration"=w379) -> (w391:refnum<class "TDMS datalogger editor node.lvclass">)
                  n193 = call <vilib>:"write engine configuration.vi"("error in"=w370, "engine configuration"=w371, "Engine Parent Editor Node in"=w386) -> ("error out"=w385:errorcluster, "Engine Parent Editor Node out"=w389:refnum<class "Engine Parent Editor Node.lvclass">)  [unwired: 7 in]
                  n194 = in-place-dvr #13(w389) -> (w367:errorcluster)  [unwired: 1 out]
                  n195 = in-place-dvr #14(w391) -> (w366:errorcluster)  [unwired: 1 out]
                }
                n196 = Merge Errors(w369, w367, w368, w366) -> (w365:errorcluster)
              }
            }
          }
        }
        n197 = case shown="Error" w91 {
          selector: w91 -> [w94 w98]
          tunnel: [w95 w99] -> w90
          tunnel: w83 -> [w95 w99]
          tunnel: [w94 w96] -> w89
          frame No Error {
          }
          frame Error {
            # "#CodeRecommended Any errors should be handled within the generating case or here. Current default is to clear everything"
            n198 = call <vilib>:"Simple Error Handler.vi"("error in (no error)"=w98) -> ("error out"=w97:errorcluster)  [unwired: 4 in, 4 out]
            n199 = call <vilib>:"Clear Errors.vi"("error in (no error)"=w97) -> ("error out"=w96:errorcluster)  [unwired: 6 in]
          }
        }
      }
    }
    frame Error {
    }
  }
  n200 = disable-structure shown="Disabled" {
    frame Disabled {
      n201 = in-place {
        in-place-border: _ -> [w408]
        in-place-border: [_] -> w395
        in-place-border: [w401] -> w396
        n202 = in-place-dvr #15() -> (w403:refnum<class "Engine Parent Editor Node.lvclass">, w404:errorcluster)  [unwired: 1 in]
        n203 = in-place-dvr #16() -> (w400:refnum<class "TDMS datalogger editor node.lvclass">, w406:errorcluster)  [unwired: 1 in]
        n204 = call <vilib>:"read engine configuration.vi"("error in"=w404, "Engine Parent Editor Node in"=w403) -> ("error out"=w399:errorcluster, "Engine Parent Editor Node out"=w402:refnum<class "Engine Parent Editor Node.lvclass">)  [unwired: 7 in, 1 out]
        n205 = Unbundle By Name(w400) -> ()  [unwired: 1 out]
        n206 = Merge Errors(w408, w399, w406) -> ()  [unwired: 1 out]
        n207 = Bundle By Name(cluster=w400) -> (w407:refnum<class "TDMS datalogger editor node.lvclass">)  [unwired: 1 in]
        n208 = call <vilib>:"write engine configuration.vi"("error in"=w399, "Engine Parent Editor Node in"=w402) -> ("error out"=w401:errorcluster, "Engine Parent Editor Node out"=w405:refnum<class "Engine Parent Editor Node.lvclass">)  [unwired: 8 in]
        n209 = in-place-dvr #15(w405) -> (w397:errorcluster)  [unwired: 1 out]
        n210 = in-place-dvr #16(w407) -> (w398:errorcluster)  [unwired: 1 out]
      }
      n211 = Merge Errors(w395, w397, w396, w398) -> ()  [unwired: 1 out]
    }
    frame Enabled {
    }
  }
  n212 = disable-structure shown="Disabled" {
    frame Disabled {
    }
    frame Enabled {
    }
  }
  n213 = Unregister For Events(event registration refnum=w36, error in=w14) -> (error out=w35:errorcluster)
  n214 = call <vilib>:"Simple Error Handler.vi"("error in (no error)"=w35) -> ()  [unwired: 4 in, 5 out]
